vi "Run Log VI.vi"(8 "error in":errorcluster, 11 "Session Handle In":T1) -> (0 "error out":errorcluster, 3 "Session Handle Out":T1)   [LabVIEW 2015, in "System Log.lvclass"]
uses:
  System Log.lvclass
  <userlib>/_Session Fwk/Typedefs/Session Handle.ctl
  <userlib>/_Session Fwk/Session - Root.lvclass
  Controls/DVR.ctl
  System Log.lvclass/System Log.ctl
  Accessors/Write Log VI.vi
  Accessors/Read Log VI.vi
  Accessors/Read UI_.vi
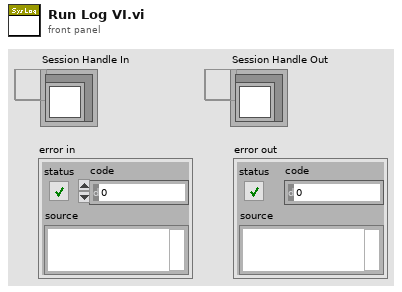
[diagram p1: front panel]
types:
  T1 = typedef "Session - Root.lvclass/Session Handle.ctl" = refnum<data-value>
  T2 = typedef "System Log.lvclass/DVR.ctl" = refnum<data-value>
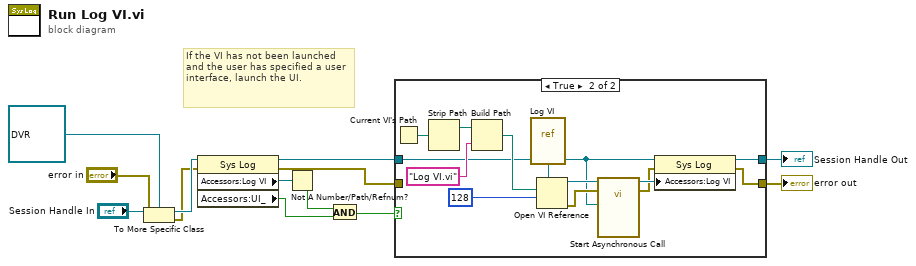
[diagram p0: block diagram]
diagram:
  # "If the VI has not been launched and the user has specified a user interface, launch the UI."
  n1 = To More Specific Class(target class=T2 refnum ("DVR"), reference="Session Handle In", error in="error in") -> (specific class reference=w8:T2, error out=w5:errorcluster)
  n2 = property class="Sys Log"(reference=w8, error in=w5) -> (reference out=w7:T2, error out=w6:errorcluster, "Accessors:Log VI"=w4:refnum<vi>, "Accessors:UI_"=w2:bool)
  n3 = Not A Number/Path/Refnum?(number/path/refnum=w4) -> (NaN/Path/Refnum?=w3:bool)
  n4 = And(x=w3, y=w2) -> (x .and. y?=w1:bool)
  n5 = case shown="True" w1 {
    tunnel: [w15 w18] -> w10
    tunnel: [w14 w17] -> w9
    tunnel: w7 -> [w15 w16]
    tunnel: w6 -> [w14 _]
    frame False {
    }
    frame True {
      n6 = Current VI's Path() -> (path=w28:path)
      n7 = Strip Path(path=w28) -> (stripped path=w27:path)  [unwired: 1 out]
      n8 = Build Path(base path=w27, name or relative path="Log VI.vi") -> (appended path=w25:path)
      n9 = vi-ref "Log VI.vi"() -> (w24:refnum<vi>)
      n10 = Open VI Reference(type specifier VI Refnum (for type only)=w24, vi path=w25, options=128) -> (vi reference=w23:refnum<vi>, error out=w22:errorcluster)  [unwired: 3 in]
      n11 = call-by-ref "Start Asynchronous Call"(reference=w23, error in=w22, "DVR"=w16) -> (reference out=w20:refnum<vi>, error out=w19:errorcluster)  [unwired: 11 in]
      n12 = property class="Sys Log"(reference=w16, error in=w19, "Accessors:Log VI"=w20) -> (reference out=w18:T2, error out=w17:errorcluster)
    }
  }
  "Session Handle Out" <- w10
  "error out" <- w9
